vi "Destroy Client.vi"(8 "error in (no error)":errorcluster, 11 "gRPC Client in":refnum<class "Template Client.lvclass">) -> (0 "error out":errorcluster, 3 "gRPC Client out":refnum<class "Template Client.lvclass">)   [LabVIEW 2019, in "Template Client.lvlib" / "Template Client.lvclass"]
uses:
  Template Client.lvclass
  Template Client.lvclass/Template Client.ctl
  <vilib>/gRPC/LabVIEW gRPC Library/gprc-lvsupport-release.lvlib
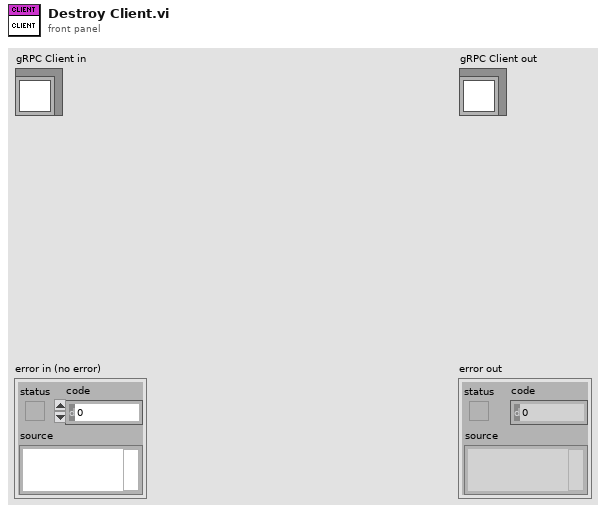
[diagram p1: front panel]
types:
  T1 = typedef "gprc-lvsupport-release.lvlib/grpcId.ctl" = u64
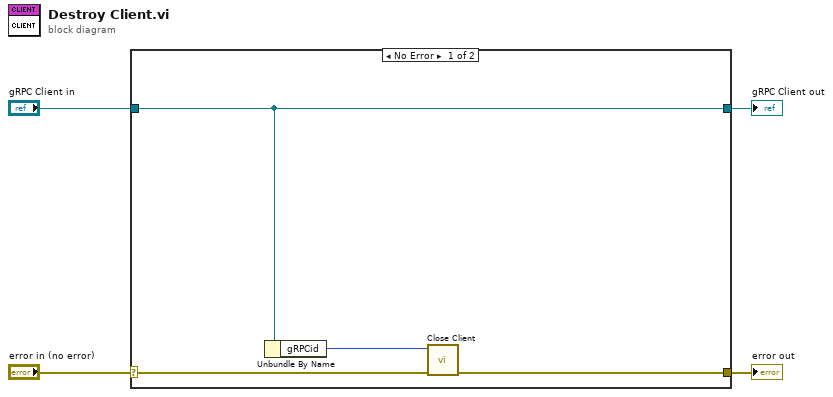
[diagram p0: block diagram]
diagram:
  n1 = case shown="No Error" "error in (no error)" {
    selector: "error in (no error)" -> [w6 w10]
    tunnel: [w5 w10] -> w3
    tunnel: [w8 w9] -> w1
    tunnel: "gRPC Client in" -> [w8 w9]
    frame No Error {
      n2 = Unbundle By Name(w8) -> ("gRPCid"=w7:T1)
      n3 = call <vilib>:"Close Client.vi"("error in (no error)"=w6, "Client Ref"=w7) -> ("error out"=w5:errorcluster)  [unwired: 9 in]
    }
    frame Error {
    }
  }
  "error out" <- w3
  "gRPC Client out" <- w1
